vi "DFS Data - Get Parent Index.vi"(8 "Error In":errorcluster, 11 "DFS Data In":T1) -> (0 "Error Out":errorcluster, 3 "Parent Index":i32)   [LabVIEW 2022 SP3]
doc: "This VI returns the \"current parent index\", i.e. the index of the parent node of the current index node."
uses:
  DFS Data (cluster).ctl
  DFS Node (cluster).ctl
  DFS Child Node (cluster).ctl
panel:
  # "Development\nControls or indicators that are useful for development or testing, but which are not outputs of the VI."
  # "Input\nInputs to the VI"
  # "Output\nOutputs of the VI"
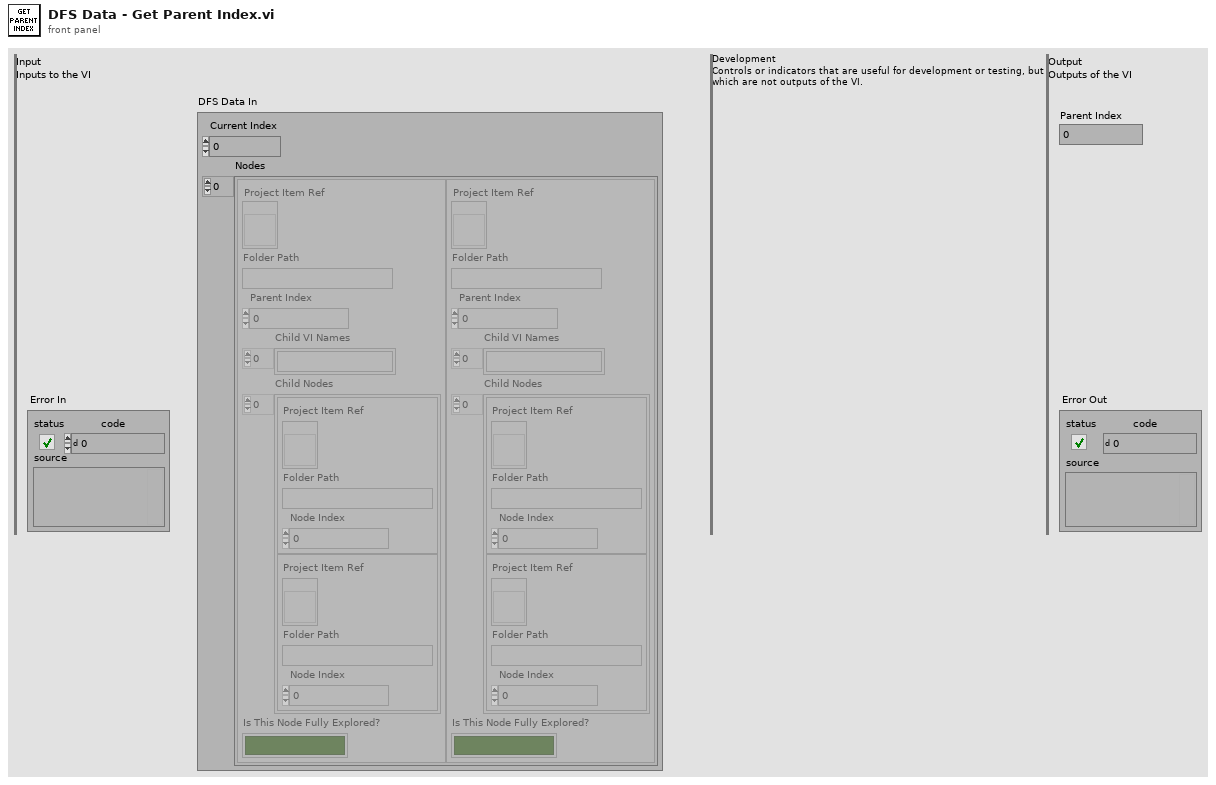
[diagram p1: front panel]
types:
  T1 = typedef "DFS Data (cluster).ctl" = cluster{"Current Index":i32, "Nodes":T2[]}
  T2 = typedef "DFS Node (cluster).ctl" = cluster{"Project Item Ref":refnum<vi>, "Folder Path":string, "Parent Index":i32, "Child VI Names":string[], "Child Nodes":T3[], "Is This Node Fully Explored?":bool}
  T3 = typedef "DFS Child Node (cluster).ctl" = cluster{"Project Item Ref":refnum<vi>, "Folder Path":string, "Node Index":i32}
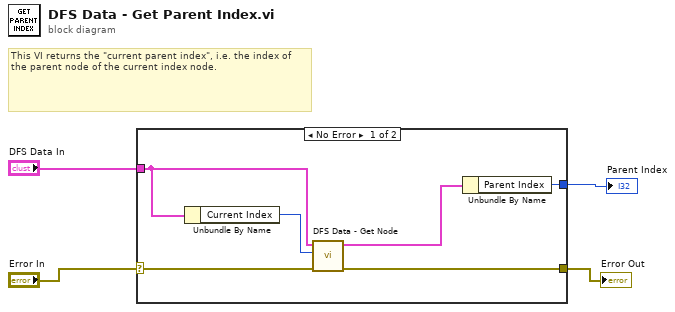
[diagram p0: block diagram]
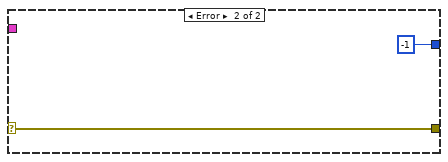
[diagram p2: hidden frame]
diagram:
  # "This VI returns the \"current parent index\", i.e. the index of the parent node of the current index node."
  n1 = case shown="No Error" "Error In" {
    selector: "Error In" -> [w10 w12]
    tunnel: [w9 w12] -> w3
    tunnel: "DFS Data In" -> [w8 _]
    tunnel: [w5 -1 ("Parent Index")] -> w1
    frame No Error {
      n2 = Unbundle By Name(w8) -> ("Current Index"=w7:i32)
      n3 = call "DFS Data - Get Node.vi"("Error In"=w10, "Node Index"=w7, "DFS Data"=w8) -> ("Error Out"=w9:errorcluster, "DFS Node"=w6:T2)  [unwired: 7 in]
      n4 = Unbundle By Name(w6) -> ("Parent Index"=w5:i32)
    }
    frame Error {
    }
  }
  "Error Out" <- w3
  "Parent Index" <- w1
